vi "tsapp_read_can_rx_buffer_datacount_win32.vi"(8 "错误输入（无错误）":errorcluster, 10 "AAppChannel":i32(ring) items=["CHN1", "CHN2", "CHN3", "CHN4", "CHN5", "CHN6", "CHN7", "CHN8", "CHN9", "CHN10", "CHN11", "CHN12", "CHN13", "CHN14", "CHN15", "CHN16", "CHN17", "CHN18", "CHN19", "CHN20", "CHN21", "CHN22", "CHN23", "CHN24", "CHN25", "CHN26", "CHN27", "CHN28", "CHN29", "CHN30", "CHN31", "CHN32"]) -> (0 "错误输出":errorcluster, 2 "AAppChannelOut":i32(ring) items=["CHN1", "CHN2", "CHN3", "CHN4", "CHN5", "CHN6", "CHN7", "CHN8", "CHN9", "CHN10", "CHN11", "CHN12", "CHN13", "CHN14", "CHN15", "CHN16", "CHN17", "CHN18", "CHN19", "CHN20", "CHN21", "CHN22", "CHN23", "CHN24", "CHN25", "CHN26", "CHN27", "CHN28", "CHN29", "CHN30", "CHN31", "CHN32"], 3 "tsapp_read_can_buffer_datacount":i32)   [LabVIEW 2016]
uses:
  TSMaster.dll
panel:
  # "功能：获取指定通道的接收报文数量"
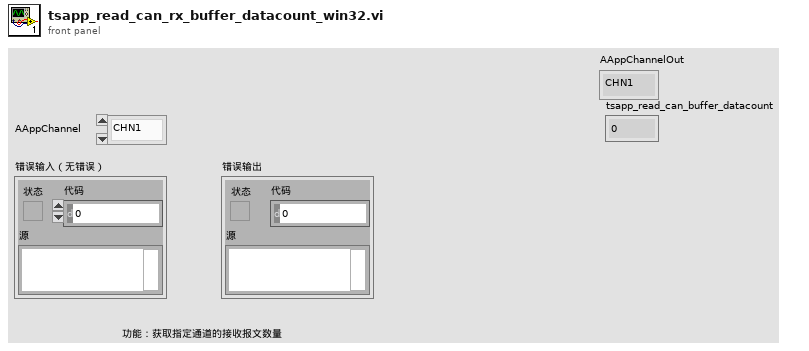
[diagram p1: front panel]
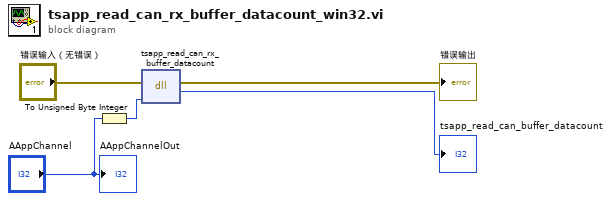
[diagram p0: block diagram]
diagram:
  n1 = To Unsigned Byte Integer(number="AAppChannel") -> (unsigned 8bit integer=w1:u8)
  n2 = dll-call lib="C:/Users/Eric/Desktop/LabVIEW/TSMasterAPI/Win32/CANopen_TS_2015/TSMaster.dll" fn="tsapp_read_can_rx_buffer_datacount"(error in="错误输入（无错误）", "AChn"=w1) -> (error out=→"错误输出":errorcluster, "tsapp_read_can_rx_buffer_datacount"=→"tsapp_read_can_buffer_datacount":i32)  [unwired: 3 in, 1 out]
  "AAppChannelOut" <- "AAppChannel"
